vi "Write bounds exp.vi"(8 "error in (no error)":errorcluster, 10 "Bounds":T1, 11 "Experiment in":refnum<class "Experiment.lvclass">) -> (0 "error out":errorcluster, 3 "Experiment out":refnum<class "Experiment.lvclass">)   [LabVIEW 2015, in "Experiment.lvclass"]
uses:
  Experiment.lvclass
  Experiment.lvclass/Experiment.ctl
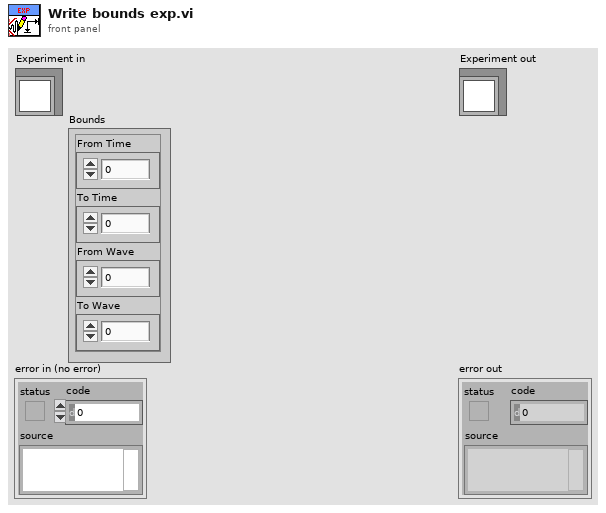
[diagram p1: front panel]
types:
  T1 = cluster{"From Time":dbl, "To Time":dbl, "From Wave":dbl, "To Wave":dbl}
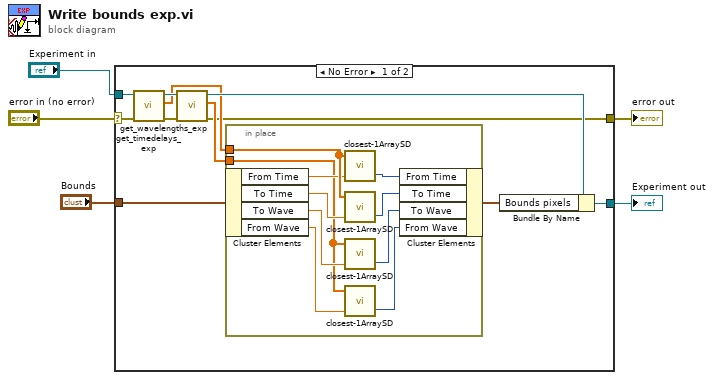
[diagram p0: block diagram]
diagram:
  n1 = case shown="No Error" "error in (no error)" {
    selector: "error in (no error)" -> [w15 w27]
    tunnel: [w6 w27] -> w4
    tunnel: [w16 w28] -> w2
    tunnel: "Experiment in" -> [w14 w28]
    tunnel: "Bounds" -> [w10 _]
    frame No Error {
      n2 = call "get_timedelays_exp.vi"("error in (no error)"=w15, "Experiment.lvclass in"=w14) -> ("error out"=w13:errorcluster, "timedelays"=w8:dbl[], "Experiment.lvclass out"=w12:refnum<class "Experiment.lvclass">)  [unwired: 7 in]
      n3 = call "get_wavelengths_exp.vi"("error in (no error)"=w13, "Experiment.lvclass in"=w12) -> ("error out"=w6:errorcluster, "wavelengths"=w7:dbl[], "Experiment.lvclass out"=w11:refnum<class "Experiment.lvclass">)  [unwired: 7 in]
      n4 = in-place {
        in-place-border: w8 -> [w26]
        in-place-border: w7 -> [w18]
        n5 = in-place-cluster #1(w10) -> ("From Time"=w23:dbl, "To Time"=w25:dbl, "To Wave"=w21:dbl, "From Wave"=w17:dbl)
        n6 = call "closest-1ArraySD.vi"("desired element"=w23, "1D Array"=w26) -> ("closest index"=w22:i32)  [unwired: 1 in, 1 out]
        n7 = call "closest-1ArraySD.vi"("desired element"=w25, "1D Array"=w26) -> ("closest index"=w24:i32)  [unwired: 1 in, 1 out]
        n8 = call "closest-1ArraySD.vi"("desired element"=w21, "1D Array"=w18) -> ("closest index"=w19:i32)  [unwired: 1 in, 1 out]
        n9 = call "closest-1ArraySD.vi"("desired element"=w17, "1D Array"=w18) -> ("closest index"=w20:i32)  [unwired: 1 in, 1 out]
        n10 = in-place-cluster #1("From Time"=w22, "To Time"=w24, "To Wave"=w19, "From Wave"=w20) -> (w9:T1)
      }
      n11 = Bundle By Name(cluster=w11, "Bounds pixels"=w9) -> (w16:refnum<class "Experiment.lvclass">)
    }
    frame Error {
    }
  }
  "error out" <- w4
  "Experiment out" <- w2
